vi "Configure Device.vi"(8 "error in (no error)":errorcluster, 10 "Max Beams":dbl, 11 "WS1050 1.1 in":refnum<class "WS1050 1.1.lvclass">) -> (0 "error out":errorcluster, 3 "WS1050 1.1 out":refnum<class "WS1050 1.1.lvclass">)   [LabVIEW 2020, in "WS1050 1.1.lvclass"]
doc: "Interface for configuring the device for testing"
uses:
  WS1050 1.1.lvclass
  Toggle 7.1.lvclass
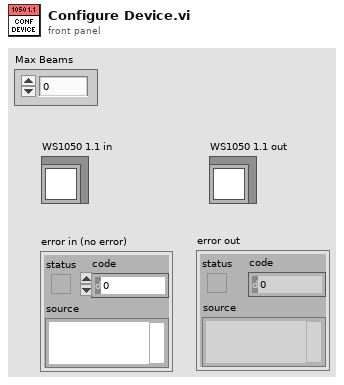
[diagram p1: front panel]
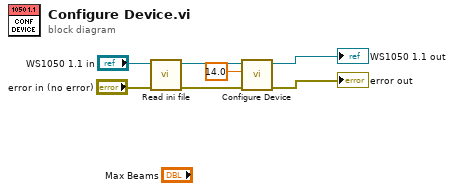
[diagram p0: block diagram]
diagram:
  n1 = call "Read ini file.vi"("Error In"="error in (no error)", "WS1050 1.1.lvclass"="WS1050 1.1 in") -> ("Error Out"=w2:errorcluster, "WS1050 1.1.lvclass Out"=w3:refnum<class "WS1050 1.1.lvclass">)  [unwired: 8 in]
  n2 = call-parent "Configure Device.vi"("error in (no error)"=w2, "Max Beams"=14.0, "Toggle 7 1.1 in"=w3) -> ("error out"=→"error out":errorcluster, "Toggle 7 1.1 out"=→"WS1050 1.1 out":refnum<class "WS1050 1.1.lvclass">)  [unwired: 7 in]
